vi "Delete String DVR.vi"(8 "error in (no error)":errorcluster, 11 "String DVR in":refnum<data-value>) -> (0 "error out":errorcluster, 3 "String out":refnum<class "String.lvclass">)   [LabVIEW 2015, in "MDSplus.lvlib" / "String.lvclass"]
uses:
  <vilib>/MDSplus/Classes/Data_Class/Scalar_Class/String_Class/String.lvclass
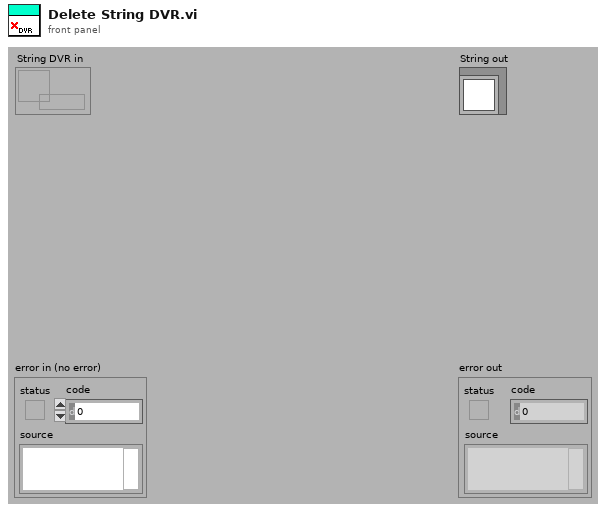
[diagram p1: front panel]
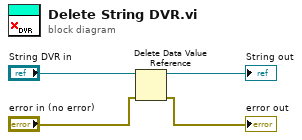
[diagram p0: block diagram]
diagram:
  n1 = Delete Data Value Reference(data value reference="String DVR in", error in="error in (no error)") -> (data value=→"String out":refnum<class "String.lvclass">, error out=→"error out":errorcluster)
